vi "StatusCmdRouting.vi"(0 "StatusVariableDataOut":T1={"DecodeMode"="Stat", "LastSerial"=0, "NoReply"=FALSE, "StatCmd"="", "StatCmdReply"="", "StatCmdReplySerial"=0, "StatusPrefix"="", "StatusData"="", "SendOut"=FALSE, "StringCmd"=FALSE, "CmdString1"="", "CmdString0"="", "Astring1"=FALSE, "CmdDataOut"="", "CmdReply"="", "CmdReplySerial"=0, "CmdArray"=[]}) -> (4 "CmdArray":u32[](array[numeric]), 6 "SendOut":bool, 8 "StringCmd":bool, 10 "CmdStringOut":string)   [LabVIEW 2020]
uses:
  TypeDefinitions/StatusVariableData.ctl
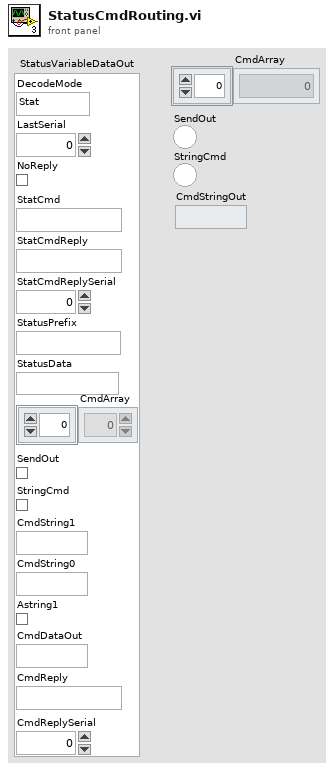
[diagram p1: front panel]
types:
  T1 = typedef "StatusVariableData.ctl" = cluster{"DecodeMode":string, "LastSerial":u32, "NoReply":bool, "StatCmd":string, "StatCmdReply":string, "StatCmdReplySerial":u32, "StatusPrefix":string, "StatusData":string, "SendOut":bool, "StringCmd":bool, "CmdString1":string, "CmdString0":string, "Astring1":bool, "CmdDataOut":string, "CmdReply":string, "CmdReplySerial":u32, "CmdArray":u32[]}
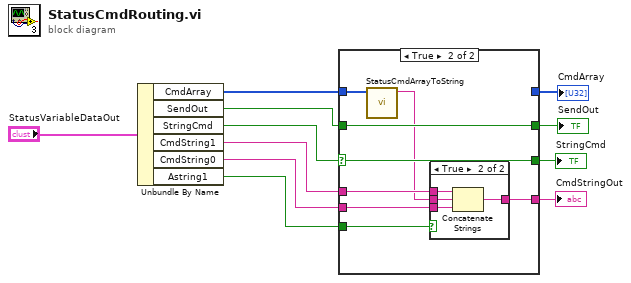
[diagram p0: block diagram]
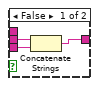
[diagram p3: hidden frame]
diagram:
  n1 = Unbundle By Name("StatusVariableDataOut") -> ("CmdArray"=w6:u32[], "SendOut"=w5:bool, "StringCmd"=w4:bool, "CmdString1"=w3:string, "CmdString0"=w2:string, "Astring1"=w1:bool)
  n2 = case shown="True" w4 {
    selector: w4 -> [w14 w21]
    tunnel: w2 -> [_ w17]
    tunnel: [w13 w22] -> w11
    tunnel: w5 -> [w13 w22]
    tunnel: [w14 w21] -> w10
    tunnel: w3 -> [_ w19]
    tunnel: [w12 _] -> w8
    tunnel: w6 -> [w12 w20]
    tunnel: [_ w16] -> w9
    tunnel: w1 -> [_ w15]
    frame False {
    }
    frame True {
      n3 = call "StatusCmdArrayToString.vi"("IncrJog"=w20) -> ("String"=w18:string)  [unwired: 10 in]
      n4 = case shown="True" w15 {
        tunnel: w19 -> [_ w29]
        tunnel: w18 -> [w25 w28]
        tunnel: w17 -> [w24 w27]
        tunnel: [w23 w26] -> w16
        frame False {
          n5 = Concatenate Strings(w25, w24) -> (w23:string)
        }
        frame True {
          n6 = Concatenate Strings(w29, w28, w27) -> (w26:string)
        }
      }
    }
  }
  "SendOut" <- w11
  "StringCmd" <- w10
  "CmdStringOut" <- w9
  "CmdArray" <- w8
